vi "Initialize.vi"(0 "Model Base in":refnum<class "Model Base.lvclass">, 11 "error in (no error)":errorcluster) -> (4 "Model Base out":refnum<class "Model Base.lvclass">, 15 "error out":errorcluster)   [LabVIEW 2023, in "Model Base.lvlib" / "Model Base.lvclass"]
uses:
  Model Base.lvclass
  Model Base.lvclass/Model Base.ctl
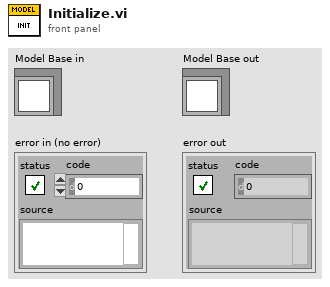
[diagram p1: front panel]
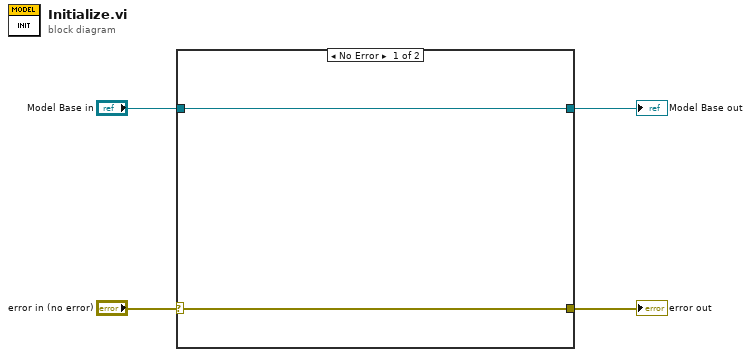
[diagram p0: block diagram]
diagram:
  n1 = case shown="No Error" "error in (no error)" {
    selector: "error in (no error)" -> [w5 w8]
    tunnel: [w5 w8] -> w3
    tunnel: [w6 w7] -> w1
    tunnel: "Model Base in" -> [w6 w7]
    frame No Error {
    }
    frame Error {
    }
  }
  "error out" <- w3
  "Model Base out" <- w1
